vi "Setup Init.vi"() -> (2 "Msg":refnum<class "Msg.lvclass">)   [LabVIEW 2021, in "jettl.lvlib" / "Setup Msg.lvlib"]
uses:
  Setup Msg.lvlib
  Msg/Msg.lvclass
  Setup Msg/Setup Msg.lvclass
  C:/git/jettl/jettl/jettl/Msg/Msg.lvclass
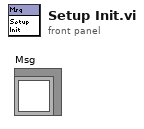
[diagram p1: front panel]
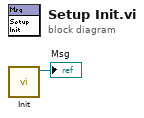
[diagram p0: block diagram]
diagram:
  n1 = call "Init.vi"() -> ("Setup Msg out"=→"Msg":refnum<class "Setup Msg.lvclass">)  [unwired: 11 in]
